vi "setUp.vi"(8 "error in (no error)":errorcluster, 11 "reference in":refnum<class "Interface Framework Single Object.lvclass">) -> (0 "error out":errorcluster, 3 "reference in":refnum<class "Interface Framework Single Object.lvclass">)   [LabVIEW 2009, in "Interface Framework Single Object.lvclass"]
doc: "setUp runs prior to the test method during test execution. Use this method to initialize any object data required by your tests."
uses:
  Interface Framework Single Object.lvclass
  Numeric Test Object/Numeric Test Object.lvclass
  Interface Framework Single Object.lvclass/Interface Framework Single Object.ctl
  <vilib>/addons/_JKI Toolkits/VI Tester/TestCase.llb/TestCase.lvclass
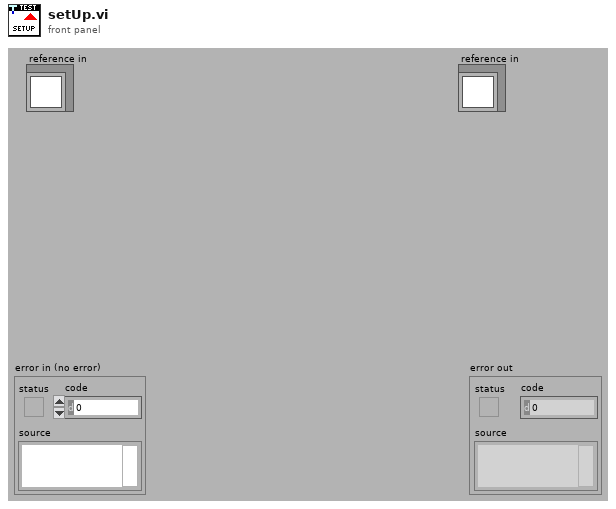
[diagram p1: front panel]
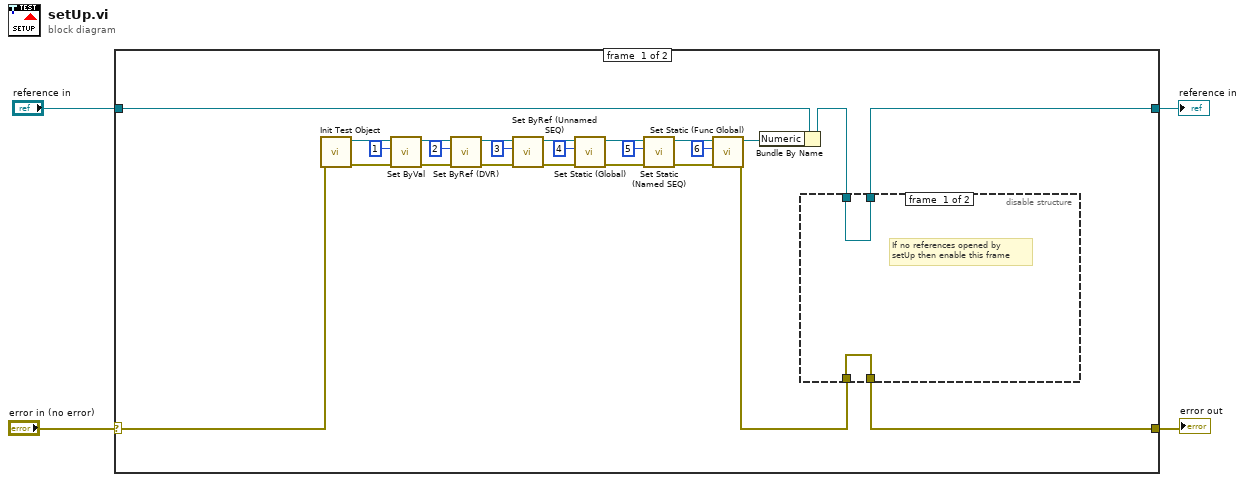
[diagram p0: block diagram]
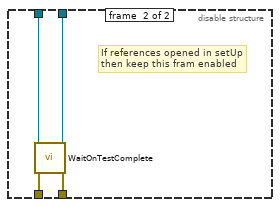
[diagram p2: hidden frame]
diagram:
  n1 = case shown="No Error" "error in (no error)" {
    selector: "error in (no error)" -> [w6 w37]
    tunnel: [w28 w37] -> w3
    tunnel: [w29 w36] -> w1
    tunnel: "reference in" -> [w27 w36]
    frame #0 {
      n2 = call "Init Test Object.vi"("error in (no error)"=w6) -> ("error out"=w5:errorcluster, "Numeric out"=w7:refnum<class "Numeric Test Object.lvclass">)  [unwired: 9 in]
      n3 = call-dynamic "Set ByVal.vi"("error in (no error)"=w5, "Int"=1, "Numeric in"=w7) -> ("error out"=w19:errorcluster, "Numeric out"=w24:refnum<class "Numeric Test Object.lvclass">)  [unwired: 7 in]
      n4 = call-dynamic "Set ByRef (DVR).vi"("error in (no error)"=w19, "Int"=2, "Numeric in"=w24) -> ("error out"=w18:errorcluster, "Numeric out"=w23:refnum<class "Numeric Test Object.lvclass">)  [unwired: 7 in]
      n5 = call-dynamic "Set ByRef (Unnamed SEQ).vi"("error in (no error)"=w18, "Int"=3, "Numeric in"=w23) -> ("error out"=w16:errorcluster, "Numeric out"=w17:refnum<class "Numeric Test Object.lvclass">)  [unwired: 7 in]
      n6 = call-dynamic "Set Static (Global).vi"("error in (no error)"=w16, "Int"=4, "Numeric in"=w17) -> ("error out"=w9:errorcluster, "Numeric out"=w14:refnum<class "Numeric Test Object.lvclass">)  [unwired: 7 in]
      n7 = call-dynamic "Set Static (Named SEQ).vi"("error in (no error)"=w9, "Int"=5, "Numeric in"=w14) -> ("error out"=w8:errorcluster, "Numeric out"=w12:refnum<class "Numeric Test Object.lvclass">)  [unwired: 7 in]
      n8 = call-dynamic "Set Static (Func Global).vi"("error in (no error)"=w8, "Int"=6, "Numeric in"=w12) -> ("error out"=w25:errorcluster, "Numeric out"=w11:refnum<class "Numeric Test Object.lvclass">)  [unwired: 7 in]
      n9 = Bundle By Name(cluster=w27, "Numeric"=w11) -> (w26:refnum<class "Interface Framework Single Object.lvclass">)
      n10 = disable-structure shown="Enabled" {
        disable-tunnel: w26 -> [w31 w35]
        disable-tunnel: [w31 w34] -> w29
        disable-tunnel: w25 -> [w30 w33]
        disable-tunnel: [w30 w32] -> w28
        frame #0 {
          # "If no references opened by\nsetUp then enable this frame"
        }
        frame #1 {
          # "If references opened in setUp\nthen keep this fram enabled"
          n11 = call <vilib>:"WaitOnTestComplete.vi"("error in (no error)"=w33, "TestCase in"=w35) -> ("error out"=w32:errorcluster, "TestCase out"=w34:refnum<class "Interface Framework Single Object.lvclass">)  [unwired: 8 in]
        }
      }
    }
    frame #1 {
    }
  }
  "error out" <- w3
  "reference in" <- w1
